vi "get missing volumes.vi"() -> ()   [LabVIEW 2024]
uses:
  <vilib>/addons/_JKI.lib/REST Client/classes/REST Client/REST Client.lvclass
  CV_RESTful_Library/CV_RESTful_Lib.lvlib
  <vilib>/addons/_JKI.lib/Serialization/JSON/JKI JSON Serialization.lvlib
panel:
  in  "stop":bool
  out "size(s)":i32
  out "progress":i32(slide) scale=0.0..15770.0
  out "missing vols out":i32[](array[numeric])
  out "URLs":string
  out "error out":errorcluster
  in  "missing vols":i32[](array[numeric])=array[7889 elements]
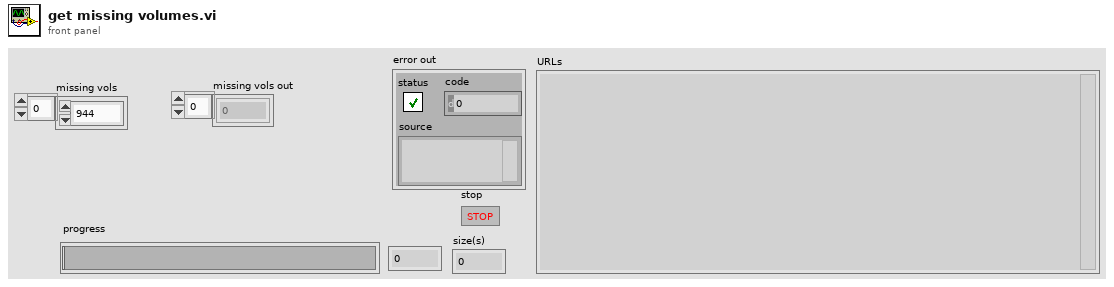
[diagram p1: front panel]
types:
  T1 = typedef "CV_RESTful_Lib.lvlib/local_volume--cluster.ctl" = cluster{"id":i32, "name":string, "sortable_name":string, "aliases":string[], "description":string, "site_detail_url":string, "count_of_issues":i32, "start_year":i32, "publisher_id":i32, "issue_ids":i32[], "date_last_updated":timestamp, "volume":i32, "cv_id":string, "volume type":T2}
  T2 = typedef "CV_Shared_Library.lvlib/volume.type--enum.ctl" = enum16{"Ongoing", "Limited Series", "Annual", "One Shot", "Reprint/Document", "Star Comics", "Epic Comics"}
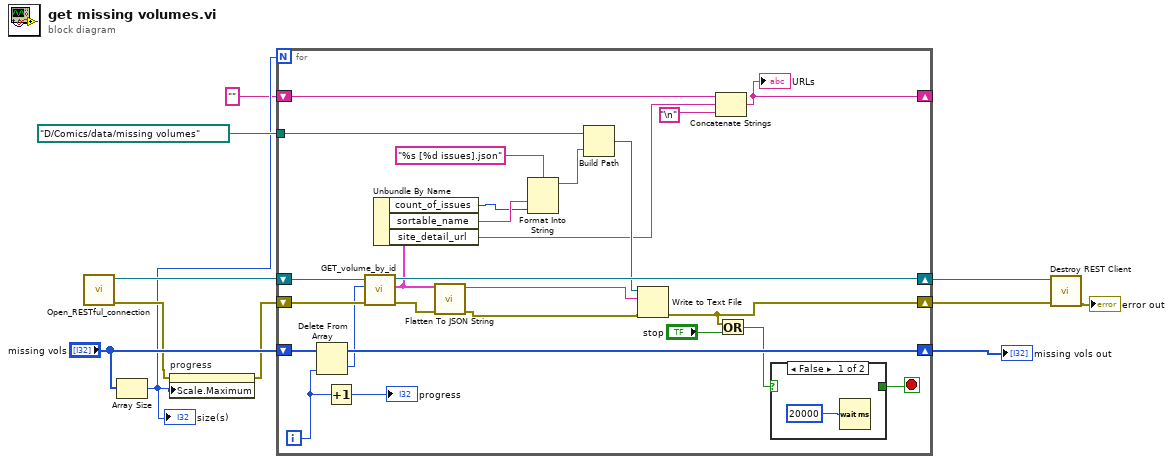
[diagram p0: block diagram]
diagram:
  n1 = call "Open_RESTful_connection.vi"() -> ("error out"=w4:errorcluster, "REST Client out"=w11:refnum<class "REST Client.lvclass">)  [unwired: 10 in]
  n2 = Array Size(array="missing vols") -> (size(s)=w2:i32)
  "size(s)" <- w2
  n3 = property on="progress" class="Slide (strict)"(error in=w4, "Scale.Maximum"=w2) -> (error out=w3:errorcluster)  [unwired: 1 in, 1 out]
  n4 = for {
    N: w2 -> [_]
    shift-right: [w18] -> w8
    shift-left: w3 -> [w37]
    shift-right: [w34] -> w10
    shift-left: w11 -> [w35]
    tunnel: path "D:/Comics/data/missing volumes" -> [w29]
    shift-right: [w23] -> w6
    shift-left: "missing vols" -> [w24]
    shift-right: [w15] -> _
    shift-left: "" -> [w17]
    i -> [w21]
    stop <- w12 stop-if-true
    n5 = Delete From Array(array=w24, index=w21) -> (deleted portion=w22:i32, array with subset deleted=w23:i32[])  [unwired: 1 in]
    n6 = Increment(x=w21) -> (x+1=→"progress":i32)
    n7 = call "GET_volume_by_id.vi"("error in (no error)"=w37, "volume id"=w22, "REST Client in"=w35) -> ("error out"=w36:errorcluster, "local volume"=w33:T1, "REST Client out"=w34:refnum<class "REST Client.lvclass">)  [unwired: 6 in]
    n8 = Unbundle By Name(w33) -> ("count_of_issues"=w30:i32, "sortable_name"=w31:string, "site_detail_url"=w16:string)
    n9 = call <vilib>:"Flatten To JSON String.vi"("error in"=w36, "Variant"=w33) -> ("error out"=w27:errorcluster, "JSON String"=w26:string)  [unwired: 8 in]
    n10 = Format Into String(format string="%s [%d issues].json", w31, w30) -> (resulting string=w25:string)  [unwired: 2 in, 1 out]
    n11 = Build Path(base path=w29, name or relative path=w25) -> (appended path=w28:path)
    n12 = Write to Text File(file (use dialog)=w28, text=w26, error in=w27) -> (error out=w18:errorcluster)  [unwired: 1 in, 2 out]
    n13 = Concatenate Strings(w17, w16, "\n") -> (w15:string)
    "URLs" <- w15
    n14 = Or(x=w18, y="stop") -> (x .or. y?=w13:bool)
    n15 = case shown="False" w13 {
      selector: w13 -> [_ w39]
      tunnel: [_ w39] -> w12
      frame False {
        n16 = Wait (ms)(milliseconds to wait=u32 20000) -> ()  [unwired: 1 out]
      }
      frame True {
      }
    }
  }
  "missing vols out" <- w6
  n17 = call-dynamic "Destroy REST Client.vi"("error in (no error)"=w8, "REST Client in"=w10) -> ("error out"=→"error out":errorcluster)  [unwired: 9 in]
